vi "Set S12CON wrapper.vi"(7 "bAckEna":i32, 8 "error in (no error)":errorcluster caption="错误输入（无错误）", 9 "pS12ConIn":T1, 10 "dwCanNodeId":u32, 11 "dwDevIndex":u32) -> (0 "error out":errorcluster caption="错误输出", 1 "pS12ConOut out":T1, 3 "function return":u32)   [LabVIEW 2016, in "UISimCanFunc_wrapper.lvlib"]
doc: "_declspec (dllexport) DWORD SetS12CON_wrapper(DWORD dwDevIndex, DWORD dwCanNodeId, P_S12CON pS12ConIn, BOOL bAckEna, P_S12CON pS12ConOut);"
uses:
  <userlib>/UISimCanFunc_wrapper/UISimCanFunc_wrapper.lvlib
  <userlib>/UISimCanFunc_wrapper/UISimCanFunc_wrapper.dll
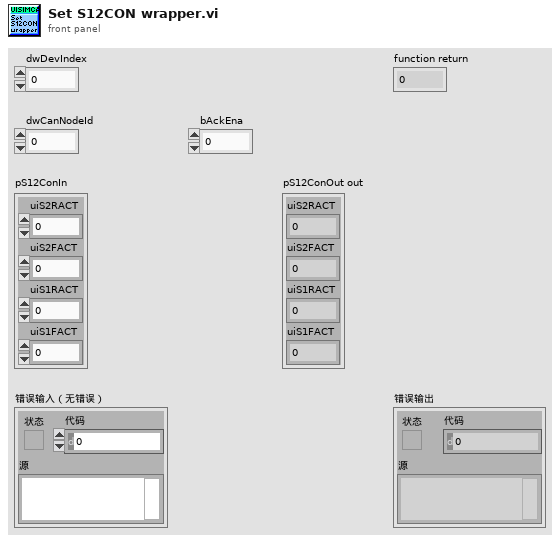
[diagram p1: front panel]
types:
  T1 = cluster{"uiS2RACT":u32, "uiS2FACT":u32, "uiS1RACT":u32, "uiS1FACT":u32}
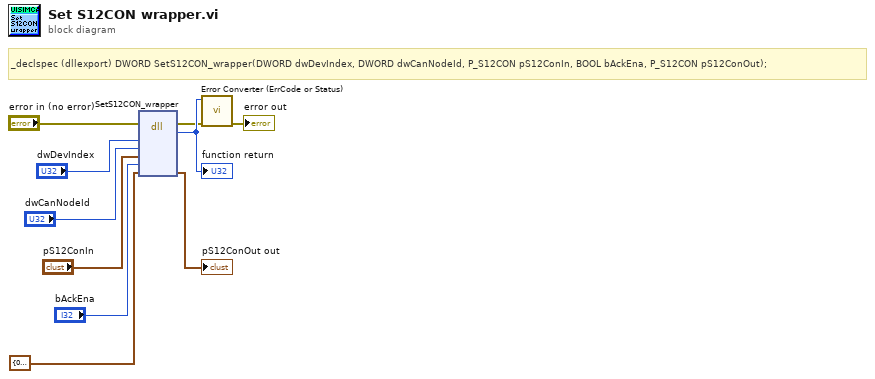
[diagram p0: block diagram]
diagram:
  # "_declspec (dllexport) DWORD SetS12CON_wrapper(DWORD dwDevIndex, DWORD dwCanNodeId, P_S12CON pS12ConIn, BOOL bAckEna, P_S12CON pS12ConOut);"
  n1 = dll-call lib="C:/Program Files (x86)/National Instruments/LabVIEW 2016/user.lib/UISimCanFunc_wrapper/UISimCanFunc_wrapper.*" fn="SetS12CON_wrapper"(error in="error in (no error)", "dwDevIndex"="dwDevIndex", "dwCanNodeId"="dwCanNodeId", "pS12ConIn"="pS12ConIn", "bAckEna"="bAckEna", "pS12ConOut"=T1 {"uiS2RACT"=0, "uiS2FACT"=0, "uiS1RACT"=0, "uiS1FACT"=0}) -> (error out=w2:errorcluster, w10:u32, "pS12ConOut"=→"pS12ConOut out":T1)  [unwired: 6 in, 1 out]
  "function return" <- w10
  n2 = call <userlib>:"Error Converter (ErrCode or Status).vi"("error in (no error)"=w2, "error code"=w10) -> ("error out"=→"error out":errorcluster)  [unwired: 9 in]
